vi "Config CDMA2000 Filter.vi"(0 "VISA Resource Name":refnum<visa-resource-name>, 1 "Filter Alpha (0.500)":dbl=0.5 format="%.3f", 2 "Filter BbT (0.500)":dbl=0.5 format="%.3f", 5 "Filter (6:IS-95 MOD w/EQ)":T1(ring)=enum."USER FIR", 7 "User FIR (FIR_DATA)":string="FIR_DATA", 9 "Optimize For (T:EVM)":bool=TRUE, 11 "error in (no error)":errorcluster {"code" format="%.0x"}) -> (4 "VISA Resource Name Out":refnum<visa-resource-name>, 15 "error out":errorcluster {"code" format="%.0x"})   [LabVIEW 2012, in "Agilent ESG Series.lvlib"]
doc: "This VI is used to configure the CDMA2000 Filter.\n\nThis VI is valid only on instruments E44xxB with the 101 option or on instrument E4438C with option 401."
uses:
  <instrlib>/Agilent ESG Series/Agilent ESG Series.lvlib
panel:
  # "EVM"
  # "ACP"
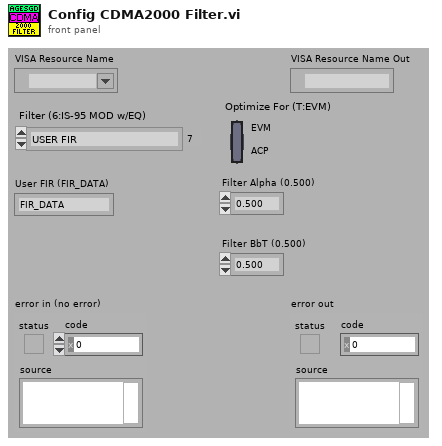
[diagram p1: front panel]
types:
  T1 = enum16{"ROOT NYQUIST", "NYQUIST", "GAUSSIAN", "IS-95", "IS-95 w/EQ", "IS-95 MOD", "IS-95 MOD w/EQ", "USER FIR", "RECTANGLE", "WCDMA", "AC4FM", "IS2000SR3DS", "UGGAUSSIAN"}
  T2 = enum16{"ROOT NYQUIST", "NYQUIST", "GAUSSIAN", "IS-95", "IS-95 w/EQ", "IS-95 MOD", "IS-95 MOD w/EQ", "USER FIR"}
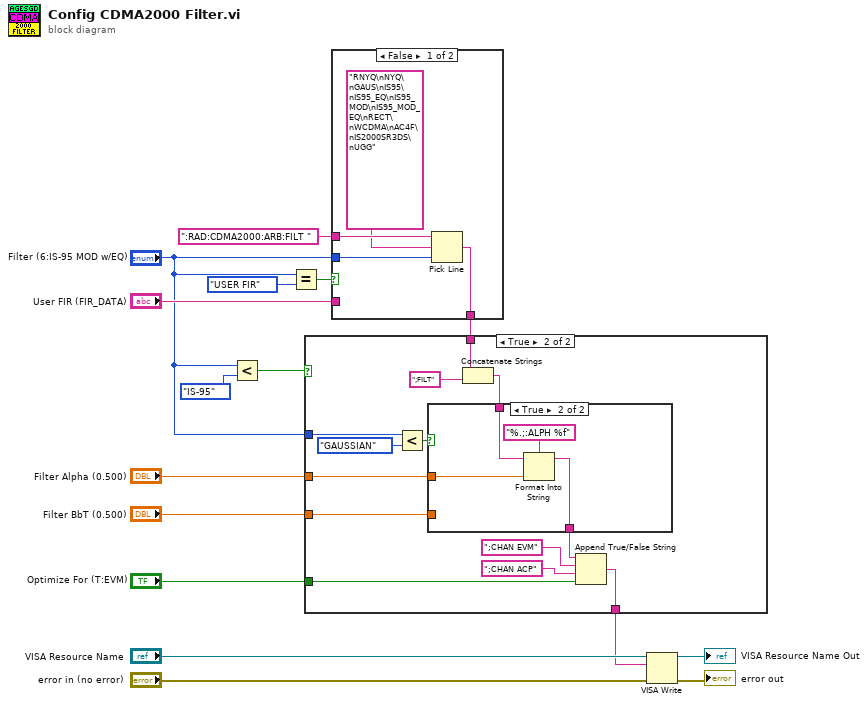
[diagram p0: block diagram]
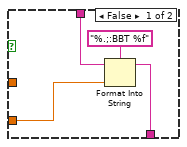
[diagram p3: hidden frame]
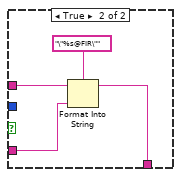
[diagram p4: hidden frame]
diagram:
  n1 = Less?(x="Filter (6:IS-95 MOD w/EQ)", y=T2."IS-95") -> (x < y?=w6:bool)
  n2 = Equal?(x="Filter (6:IS-95 MOD w/EQ)", y=T2."USER FIR") -> (x = y?=w10:bool)
  n3 = case shown="False" w10 {
    tunnel: ":RAD:CDMA2000:ARB:FILT " ("string (\"\")") -> [w20 w24]
    tunnel: "Filter (6:IS-95 MOD w/EQ)" -> [w18 _]
    tunnel: [w17 w22] -> w5
    tunnel: "User FIR (FIR_DATA)" -> [_ w21]
    frame False {
      n4 = Pick Line(string ("")=w20, multi-line string="RNYQ\nNYQ\nGAUS\nIS95\nIS95_EQ\nIS95_MOD\nIS95_MOD_EQ\nRECT\nWCDMA\nAC4F\nIS2000SR3DS\nUGG", line index=w18) -> (output string=w17:string)
    }
    frame True {
      n5 = Format Into String(format string="\"%s@FIR\"", initial string=w24, w21) -> (resulting string=w22:string)  [unwired: 1 in, 1 out]
    }
  }
  n6 = case shown="True" w6 {
    tunnel: "Optimize For (T:EVM)" -> [_ w38]
    tunnel: [w25 w31] -> w1
    tunnel: w5 -> [w25 w28]
    tunnel: "Filter (6:IS-95 MOD w/EQ)" -> [_ w36]
    tunnel: "Filter BbT (0.500)" -> [_ w30]
    tunnel: "Filter Alpha (0.500)" -> [_ w29]
    frame False {
    }
    frame True {
      n7 = Less?(x=w36, y=T2."GAUSSIAN") -> (x < y?=w35:bool)
      n8 = Concatenate Strings(w28, ";FILT") -> (w26:string)
      n9 = case shown="True" w35 {
        tunnel: w26 -> [w41 w45]
        tunnel: [w40 w44] -> w32
        tunnel: w30 -> [w39 _]
        tunnel: w29 -> [_ w43]
        frame False {
          n10 = Format Into String(format string="%.;:BBT %f", initial string=w41, w39) -> (resulting string=w40:string)  [unwired: 1 in, 1 out]
        }
        frame True {
          n11 = Format Into String(format string="%.;:ALPH %f", initial string=w45, w43) -> (resulting string=w44:string)  [unwired: 1 in, 1 out]
        }
      }
      n12 = Append True/False String(1:w38, 2:";CHAN ACP" ("false string"), 3:";CHAN EVM" ("false string"), 4:w32) -> (0:w31:string)
    }
  }
  n13 = VISA Write(VISA resource name="VISA Resource Name", write buffer=w1, error in (no error)="error in (no error)") -> (VISA resource name out=→"VISA Resource Name Out":refnum<visa-resource-name>, error out=→"error out":errorcluster)  [unwired: 1 out]
